vi "Drive Controller.vi"(8 "error in":errorcluster) -> ()   [LabVIEW 2020]
doc: "This VI executes continuously carrying out the current operation and responding to updates or new operation requests. It will often contain the timing or control code that is difficult to place directly in TeleOp. This VI generally opens all sensors and motors and isolates the rest of the robot code from knowing implementation details of how the operations are carried out."
uses:
  <vilib>/Rock Robotics/WPI/Framework/Completion Status.ctl
  Drive Setpoints.ctl
  Drive Operations.ctl
  <vilib>/Rock Robotics/WPI/SafetyOutput/WPI_SafetyOutputConfigMenu.ctl
  <vilib>/Rock Robotics/WPI/RobotDrive/WPI_RobotDriveOpen2MotorWithExistingMotors.vi
  <vilib>/Rock Robotics/Network Tables/NT Write Number.vi
  <vilib>/Rock Robotics/Network Tables/NT Write Variant.vi
panel:
  in  "Interactive Values":T1
  in  "Buttons":cluster{"Execute Cmd":bool, "Abort Cmd":bool}
  out "Command Timing":cluster{"Start Time (ms)":u32, "Iterations":i32}
  out "Status":T3
  out "Setpoints":T4(graph)
  out "Current\nCmd":string
  # "Tip: The graph shows the motor setpoints. It may also be helpful to observe inputs and sensor values.\nYou may also want to display tuning or debugging controls."
  # "Interactive Command: You may fill in the settings for a command\nand schedule it with the Execute button. You can observe and abort\nany command while fine tuning the code for the controller."
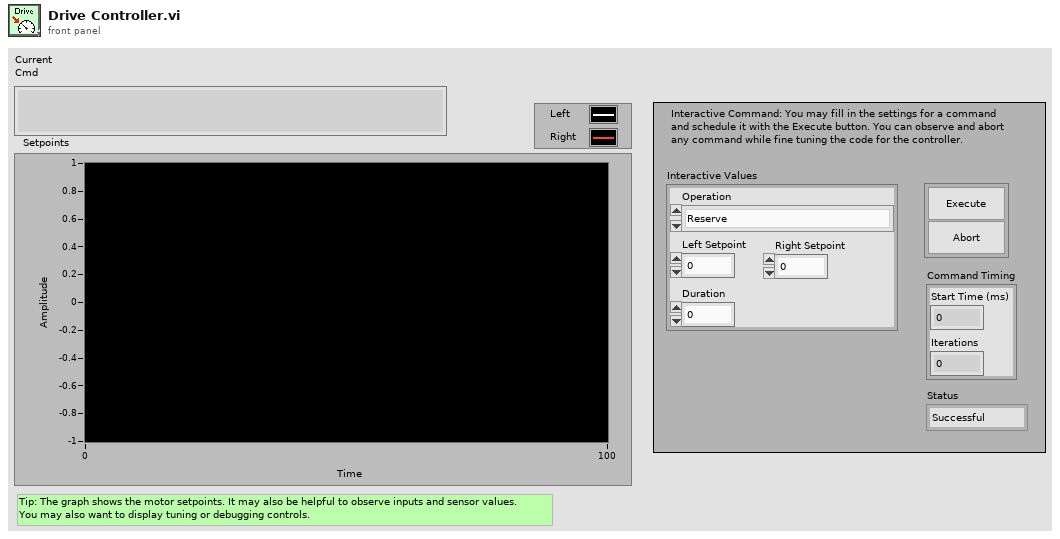
[diagram p1: front panel]
types:
  T1 = typedef "Drive Setpoints.ctl" = cluster{"Operation":T2, "Left Setpoint":dbl, "Right Setpoint":dbl, "Duration":dbl}
  T2 = typedef "Drive Operations.ctl" = enum16{"Reserve", "Read Current", "Immediate", "Drive for Time", "Drive for Distance"}
  T3 = typedef "Completion Status.ctl" = enum16{"Successful", "Aborted", "Incomplete"}
  T4 = cluster{"Left Setpoint":dbl, "Right Setpoint":dbl}
  T5 = typedef "WPI_SafetyOutputConfigMenu.ctl" = enum16{"Enable", "Disable"}
  T6 = typedef "WPI_MotorControlDeviceRef.ctl" = cluster{"DeviceStatus":errorcluster, "Type":T7, "PWM":cluster{"PWM Channel":T8, "DeadBand":T9}, "CAN":cluster{"Device Number":u8, "SetOutput VI Ref":variant, "GetOutput VI Ref":variant, "Enable VI Ref":variant, "Disable VI Ref":variant, "Data":variant}, "Invert":bool, "DIO PWM":cluster{"PWM \"Enable\" Channel":T8, "DIOChannel":T10, "PWM Rate":dbl}}
  T7 = typedef "WPI_MotorControlType.ctl" = enum16{"PWM", "CAN", "DIO PWM"}
  T8 = typedef "FPGA_DIOPWMChannel.ctl" = enum8{"PWM 0", "PWM 1", "PWM 2", "PWM 3", "PWM 4", "PWM 5", "PWM 6", "PWM 7", "PWM 8", "PWM 9", "PWM MXP 0", "PWM MXP 1", "PWM MXP 2", "PWM MXP 3", "PWM MXP 4", "PWM MXP 5", "PWM MXP 6", "PWM MXP 7", "PWM MXP 8", "PWM MXP 9", "Invalid"}
  T9 = typedef "WPI_PWMDeadband.ctl" = cluster{"Name":string, "maxPositivePwm":i32, "minPositivePwm":i32, "centerPwm":i32, "maxNegativePwm":i32, "minNegativePwm":i32, "angularRange":u16}
  T10 = typedef "FPGA_DIOChannel.ctl" = enum8{"DIO 0", "DIO 1", "DIO 2", "DIO 3", "DIO 4", "DIO 5", "DIO 6", "DIO 7", "DIO 8", "DIO 9", "DIO MXP 0", "DIO MXP 1", "DIO MXP 2", "DIO MXP 3", "DIO MXP 4", "DIO MXP 5", "DIO MXP 6", "DIO MXP 7", "DIO MXP 8", "DIO MXP 9", "DIO MXP 10", "DIO MXP 11", "DIO MXP 12", "DIO MXP 13", "DIO MXP 14", "DIO MXP 15", "SPI Port CS1", "SPI Port CS2", "SPI Port CS3", "SPI Port MISO", "SPI Port MOSI", "Invalid"}
  T11 = typedef "WPI_RobotDriveDevRef.ctl" = cluster{"DevStatus":errorcluster, "Motors[]":T6[], "Square Inputs":bool, "Max Output":dbl}
  T12 = typedef "Command Status Info.ctl" = cluster{"Name":string, "Status":T3, "notifier out":T13}
  T13 = typedef "Completion Notifier.ctl" = refnum<notifier>
  T14 = cluster{"SubSystem Data":T1, cluster{"Start Time (ms)":u32, "Iterations":i32}, cluster{"Command Info":T12, "Description":string, "Default Command":T1, "queue out":refnum<queue>, "Subsystem Name":string}}
  T15 = cluster{"SubSystem Data":T1, cluster{"Start Time (ms)":u32, "Iterations":i32}, "Default Command Arguments":cluster{"Command Info":T12, "Description":string, "Default Command":T1, "queue out":refnum<queue>, "Subsystem Name":string}}
  T16 = cluster{"Don't move motors while reserved":dbl, "Don't move motors while reserved":dbl}
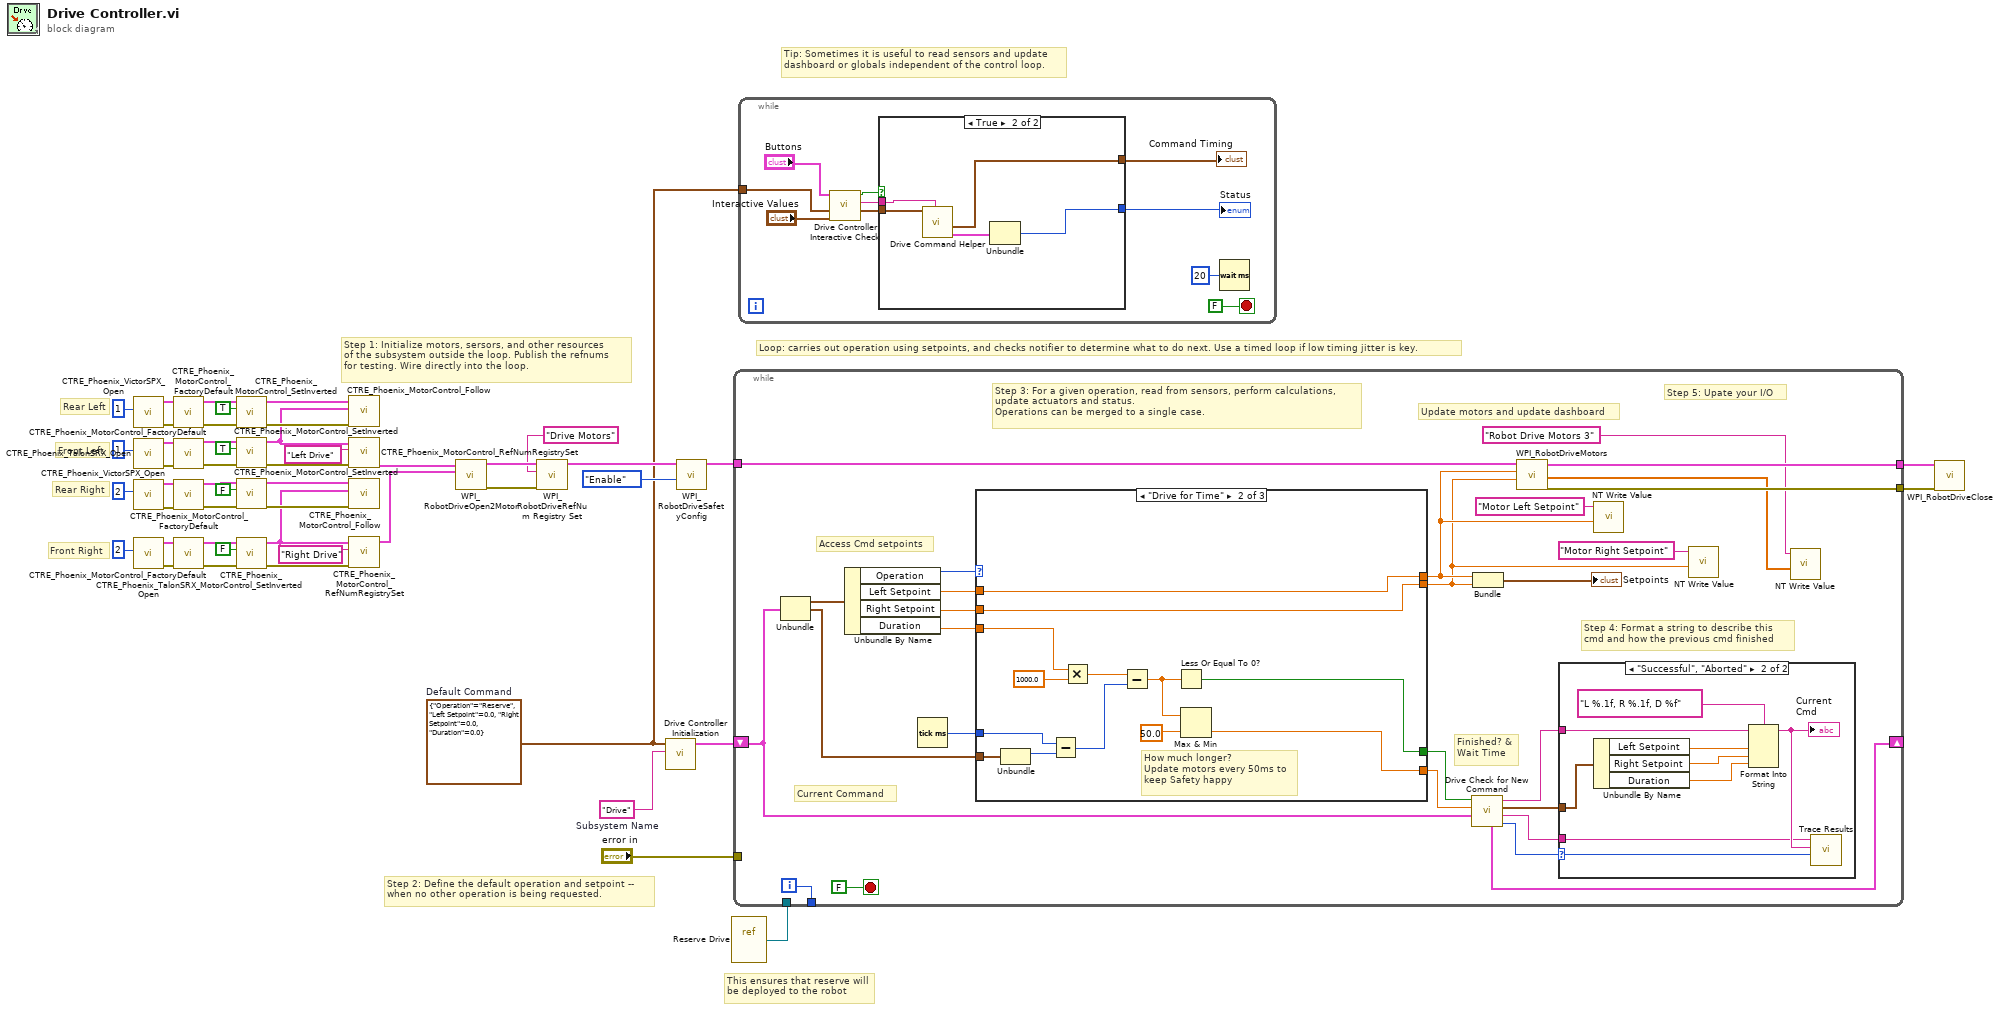
[diagram p0: block diagram]
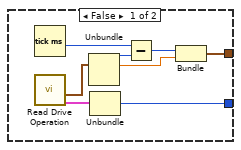
[diagram p2: hidden frame]
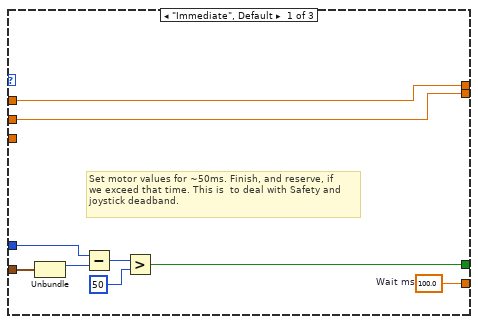
[diagram p4: hidden frame]
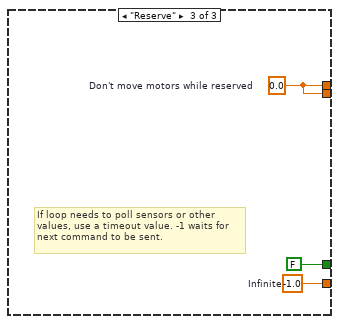
[diagram p5: hidden frame]
diagram:
  w39 = T1 {"Operation"=enum."Reserve", "Left Setpoint"=0.0, "Right Setpoint"=0.0, "Duration"=0.0}  # Default Command
  w49 = "Drive"  # Subsystem Name
  # "Front Right"
  # "Front Left"
  # "Rear Right"
  # "Rear Left"
  # "This ensures that reserve will\nbe deployed to the robot"
  # "Tip: Sometimes it is useful to read sensors and update\ndashboard or globals independent of the control loop."
  # "Step 2: Define the default operation and setpoint --\nwhen no other operation is being requested."
  # "Step 1: Initialize motors, sersors, and other resources\nof the subsystem outside the loop. Publish the refnums\nfor testing. Wire directly into the loop."
  # "Loop: carries out operation using setpoints, and checks notifier to determine what to do next. Use a timed loop if low timing jitter is key."
  n1 = call <vilib>:"CTRE_Phoenix_VictorSPX_Open.vi"("Device Number"=u8 1) -> ("error out"=w32:errorcluster, "PhoenixMotorControlDevRef"=w31:T6)  [unwired: 9 in]
  n2 = call <vilib>:"CTRE_Phoenix_TalonSRX_Open.vi"("Device Number"=u8 1) -> ("error out"=w29:errorcluster, "PhoenixMotorControlDevRef"=w30:T6)  [unwired: 9 in]
  n3 = call <vilib>:"CTRE_Phoenix_VictorSPX_Open.vi"("Device Number"=u8 2) -> ("error out"=w28:errorcluster, "PhoenixMotorControlDevRef"=w27:T6)  [unwired: 9 in]
  n4 = call <vilib>:"CTRE_Phoenix_TalonSRX_Open.vi"("Device Number"=u8 2) -> ("error out"=w26:errorcluster, "PhoenixMotorControlDevRef"=w25:T6)  [unwired: 9 in]
  n5 = call <vilib>:"CTRE_Phoenix_MotorControl_FactoryDefault.vi"("error in"=w32, "PhoenixMotorControlDevRef"=w31) -> ("error out"=w23:errorcluster, "PhoenixMotorControlDevRef"=w22:T6)  [unwired: 8 in]
  n6 = call <vilib>:"CTRE_Phoenix_MotorControl_FactoryDefault.vi"("error in"=w29, "PhoenixMotorControlDevRef"=w30) -> ("error out"=w17:errorcluster, "PhoenixMotorControlDevRef"=w18:T6)  [unwired: 8 in]
  n7 = call <vilib>:"CTRE_Phoenix_MotorControl_FactoryDefault.vi"("error in"=w28, "PhoenixMotorControlDevRef"=w27) -> ("error out"=w13:errorcluster, "PhoenixMotorControlDevRef"=w12:T6)  [unwired: 8 in]
  n8 = call <vilib>:"CTRE_Phoenix_MotorControl_FactoryDefault.vi"("error in"=w26, "PhoenixMotorControlDevRef"=w25) -> ("error out"=w8:errorcluster, "PhoenixMotorControlDevRef"=w7:T6)  [unwired: 8 in]
  n9 = call <vilib>:"CTRE_Phoenix_MotorControl_SetInverted.vi"("error in (no error)"=w23, "Invert?"=TRUE, "PhoenixMotorControlDevRef"=w22) -> ("error out"=w20:errorcluster, "PhoenixMotorControlDevRef"=w21:T6)  [unwired: 7 in]
  n10 = call <vilib>:"CTRE_Phoenix_MotorControl_SetInverted.vi"("error in (no error)"=w17, "Invert?"=TRUE, "PhoenixMotorControlDevRef"=w18) -> ("error out"=w16:errorcluster, "PhoenixMotorControlDevRef"=w15:T6)  [unwired: 7 in]
  n11 = call <vilib>:"CTRE_Phoenix_MotorControl_SetInverted.vi"("error in (no error)"=w13, "Invert?"=FALSE, "PhoenixMotorControlDevRef"=w12) -> ("error out"=w10:errorcluster, "PhoenixMotorControlDevRef"=w11:T6)  [unwired: 7 in]
  n12 = call <vilib>:"CTRE_Phoenix_MotorControl_SetInverted.vi"("error in (no error)"=w8, "Invert?"=FALSE, "PhoenixMotorControlDevRef"=w7) -> ("error out"=w5:errorcluster, "PhoenixMotorControlDevRef"=w6:T6)  [unwired: 7 in]
  n13 = call <vilib>:"CTRE_Phoenix_MotorControl_Follow.vi"("error in (no error)"=w20, "Master Controller to Follow"=w15, "PhoenixMotorControlDevRef"=w21) -> ()  [unwired: 7 in, 2 out]
  n14 = call <vilib>:"CTRE_Phoenix_MotorControl_RefNumRegistrySet.vi"("error in (no error)"=w16, "refnum name"="Left Drive", "PhoenixMotorControlDevRef"=w15) -> ("PhoenixMotorControlDevRef"=w4:T6)  [unwired: 7 in, 1 out]
  n15 = call <vilib>:"CTRE_Phoenix_MotorControl_Follow.vi"("error in (no error)"=w10, "Master Controller to Follow"=w6, "PhoenixMotorControlDevRef"=w11) -> ()  [unwired: 7 in, 2 out]
  n16 = call <vilib>:"CTRE_Phoenix_MotorControl_RefNumRegistrySet.vi"("error in (no error)"=w5, "refnum name"="Right Drive", "PhoenixMotorControlDevRef"=w6) -> ("PhoenixMotorControlDevRef"=w3:T6)  [unwired: 7 in, 1 out]
  n17 = call-poly <vilib>:"WPI_RobotDriveOpen2Motor.vi"("Right Motor Dev Ref"=w3, "Left Motor Dev Ref"=w4) -> ("error out"=w46:errorcluster, "RobotDriveDevRef"=w48:T11)  [unwired: 3 in, 5 out]
  n18 = call <vilib>:"WPI_RobotDriveRefNum Registry Set.vi"("error in (no error)"=w46, "refnum name"="Drive Motors", "RobotDriveDevRef"=w48) -> ("RobotDriveDevRef"=w45:T11)  [unwired: 1 in, 7 out]
  n19 = call "Drive Controller Initialization.vi"("Subsystem Name"=w49, "Default Command"=w39) -> ("Current Command"=w41:T14)  [unwired: 9 in]
  n20 = call <vilib>:"WPI_RobotDriveSafetyConfig.vi"("mode"=WPI_SafetyOutputConfigMenu."Enable", "RobotDriveDevRef"=w45) -> ("RobotDriveDevRef"=w43:T11)  [unwired: 8 in, 1 out]
  n21 = vi-ref "Reserve Drive.vi"() -> (w40:refnum<vi>)
  n22 = while {
    shift-right: [w65] -> _
    shift-left: w41 -> [w58]
    tunnel: [w75] -> _
    tunnel: w43 -> [w73]
    tunnel: "error in" -> [_]
    tunnel: w40 -> [_]
    tunnel: [w57] -> w2
    tunnel: [w56] -> w1
    i -> [w75]
    stop <- FALSE stop-if-true
    # "Step 5: Upate your I/O"
    # "Step 4: Format a string to describe this\ncmd and how the previous cmd finished"
    # "Current Command"
    # "Update motors and update dashboard"
    # "Access Cmd setpoints"
    # "Finished? &\nWait Time"
    # "Step 3: For a given operation, read from sensors, perform calculations,\nupdate actuators and status.\nOperations can be merged to a single case."
    n23 = Unbundle(w58) -> ("SubSystem Data"=w72:T1, w59:cluster{"Start Time (ms)":u32, "Iterations":i32})  [unwired: 1 out]
    n24 = Unbundle By Name(w72) -> ("Operation"=w71:T2, "Left Setpoint"=w70:dbl, "Right Setpoint"=w69:dbl, "Duration"=w68:dbl)
    n25 = Tick Count (ms)() -> (millisecond timer value=w67:u32)
    n26 = case shown="\"Drive for Time\"" w71 {
      tunnel: [w94 w95 w110] -> w64
      tunnel: [w87 w102 FALSE ("ignore previous (F)")] -> w63
      tunnel: w59 -> [w86 w104 _]
      tunnel: [w93 w101 w108] -> w51
      tunnel: [w92 w100 w108] -> w50
      tunnel: w70 -> [w93 w101 _]
      tunnel: w69 -> [w92 w100 _]
      tunnel: w68 -> [_ w99 _]
      tunnel: w67 -> [w88 w98 _]
      frame "Immediate", Default {
        w94 = 100.0  # Wait ms
        # "Set motor values for ~50ms. Finish, and reserve, if\nwe exceed that time. This is  to deal with Safety and\njoystick deadband."
        n27 = Unbundle(w86) -> ("Start Time (ms)"=w89:u32)  [unwired: 1 out]
        n28 = Subtract(x=w88, y=w89) -> (x-y=w90:u32)
        n29 = Greater?(x=w90, y=u8 50 ("Left Motor")) -> (0:w87:bool)
      }
      frame "Drive for Time" {
        # "How much longer?\nUpdate motors every 50ms to\nkeep Safety happy"
        n30 = Unbundle(w104) -> ("Start Time (ms)"=w103:u32)  [unwired: 1 out]
        n31 = Subtract(x=w98, y=w103) -> (x-y=w107:u32)
        n32 = Multiply(x=w99, y=1000.0) -> (x*y=w106:dbl)
        n33 = Subtract(x=w106, y=w107) -> (x-y=w97:dbl)
        n34 = Less Or Equal To 0?(x=w97) -> (x <= 0?=w102:bool)
        n35 = Max & Min(x=w97, y=50.0) -> (min(x,y)=w95:dbl)  [unwired: 1 out]
      }
      frame "Reserve" {
        w108 = 0.0  # Don't move motors while reserved
        w110 = -1.0  # Infinite
        # "If loop needs to poll sensors or other\nvalues, use a timeout value. -1 waits for\nnext command to be sent."
      }
    }
    n36 = call "Drive Check for New Command.vi"("input cluster"=w58, "Wait time (ms)"=w64, "Finished?"=w63) -> ("Completion"=w66:T3, "Subsystem Name"=w60:string, "Current Command"=w61:T1, "Initial Trace String"=w62:string, "Next Command"=w65:T15)  [unwired: 4 in]
    n37 = Bundle("Don't move motors while reserved"=w51, "Don't move motors while reserved"=w50) -> (→"Setpoints":T16)  [unwired: 1 in]
    n38 = call <vilib>:"WPI_RobotDriveMotors.vi"("RightSpeed"=w50, "LeftSpeed"=w51, "RobotDriveDevRef"=w73) -> ("error out"=w56:errorcluster, "Motor Values"=w54:dbl[], "RobotDriveDevRef"=w57:T11)  [unwired: 1 in, 5 out]
    n39 = case shown="\"Successful\", \"Aborted\"" w66 {
      selector: w66 -> [_ w85]
      tunnel: w62 -> [_ w80]
      tunnel: w61 -> [_ w81]
      tunnel: w60 -> [_ w77]
      frame "Incomplete", Default {
        # "Continuing current command"
      }
      frame "Successful", "Aborted" {
        # "Report and setup for next command"
        n40 = Unbundle By Name(w81) -> ("Left Setpoint"=w83:dbl, "Right Setpoint"=w84:dbl, "Duration"=w78:dbl)
        n41 = Format Into String(format string="L %.1f, R %.1f, D %f", initial string=w80, w83, w84, w78) -> (resulting string=w79:string)  [unwired: 1 in, 1 out]
        "Current\nCmd" <- w79
        n42 = call <vilib>:"Trace Results.vi"("Status of previous command"=w85, "Description"=w79, "Subsystem"=w77) -> ()  [unwired: 9 in]
      }
    }
    n43 = call-poly <vilib>:"NT Write Value.vi"("Numeric"=w51, "Name"="Motor Left Setpoint") -> ()  [unwired: 9 in, 1 out]
    n44 = call-poly <vilib>:"NT Write Value.vi"("Numeric"=w50, "Name"="Motor Right Setpoint") -> ()  [unwired: 9 in, 1 out]
    n45 = call-poly <vilib>:"NT Write Value.vi"("Variant"=w54, "Name"="Robot Drive Motors 3") -> ()  [unwired: 9 in, 1 out]
  }
  n46 = while {
    tunnel: w39 -> [w112]
    stop <- FALSE stop-if-true
    n47 = call "Drive Controller Interactive Check.vi"("Interactive Command In"="Interactive Values", "Default Command"=w112, "Buttons"="Buttons") -> ("Interactive Command Out"=w114:T1, "Trace String"=w115:string, "Schedule"=w116:bool)  [unwired: 6 in]
    n48 = case shown="True" w116 {
      tunnel: [w125 w133] -> w117
      tunnel: [w124 w129] -> w118
      tunnel: w115 -> [_ w131]
      tunnel: w114 -> [_ w130]
      frame False {
        n49 = Tick Count (ms)() -> (millisecond timer value=w128:u32)
        n50 = call "Read Drive Operation.vi"() -> ("Command Info"=w122:T12, "SubSystem Data"=w121:T1)  [unwired: 9 in, 1 out]
        n51 = Unbundle(w121) -> ("Operation"=w126:T2, "Left Setpoint"=w123:dbl)  [unwired: 2 out]
        n52 = Unbundle(w122) -> ("Status"=w125:T3)  [unwired: 2 out]
        n53 = Subtract(x=w128, y=w126) -> (x-y=w127:u32)
        n54 = Bundle(w127, "Left Setpoint"=w123) -> (w124:cluster{u32, "Left Setpoint":dbl})  [unwired: 1 in]
      }
      frame True {
        n55 = call "Drive Command Helper.vi"("Description"=w131, "SubSystem Data"=w130) -> ("Command Info Out"=w132:T12, "Command Timing"=w129:cluster{"Start Time (ms)":u32, "Iterations":i32})  [unwired: 7 in, 1 out]
        n56 = Unbundle(w132) -> ("Status"=w133:T3)  [unwired: 2 out]
      }
    }
    "Status" <- w117
    "Command Timing" <- w118
    n57 = Wait (ms)(milliseconds to wait=u32 20) -> ()  [unwired: 1 out]
  }
  n58 = call <vilib>:"WPI_RobotDriveClose.vi"("error in (no error)"=w1, "RobotDriveDevRef"=w2) -> ()  [unwired: 9 in, 1 out]
